vi "UI_uncorrupted.vi"() -> ()   [LabVIEW 2012]
doc: "Host interface for communication with CRD and PAS. This application currently must be running before the servers (PAS and CRD chassis) are running). At startup, the host will poll the LAN for a UDP connection to each instrument, pinging on port 5555. The acquisition loop will configure the FP and then move into a waiting state where it is polling for a connection on TCP/IP using the STM Connection Manager. When one of the instruments responds to the host, a new TCP connection will be opened on port 5556 and added to the connection manager. Seeing the connection, this VI will move from a wait state to the acquisition state where connections will be monitored. \n\nDuring the acquisition state, the host will handle messages sent via TCP/IP from the instruments. A queued state machine will determine how the data packets sent from the different instruments is handled."
uses:
  Interface/Controls/Host_State.ctl
  <vilib>/real-time/NI_Real-Time Libraries.lvlib
  Reusable/Xctls/Buffer/2D Control/2D Buffer Display.xctl
  Interface/CRDS/tau_state.ctl
  <vilib>/real-time/rtutility.llb/RT Restart Target (IP).vi
  Interface/Controls/PAS_MFC_SP.ctl
  Reusable/File IO/File Utilities.lvlib
  <userlib>/_JGCODE/error_logger/_error_logger.llb/ErrorLogger.lvclass
  Interface/CRDS/Controls/Ringdown Xctl/Ringdown.xctl
  Data/cPAS Cell Data/cPAS Cell Data.lvclass
  Data/cPAS Data.lvclass
  CRDS/Data/cCRDS Data.lvclass
  Reusable/PAS/Data/Cell/PAS Cell Data.lvclass
  Reusable/CRDS/Data/Cell/CRDS Cell Data.lvclass
  Interface/Controls/pasCellTEC.ctl
  Interface/Controls/pasTECen.ctl
  Interface/Controls/pasLasCtl.ctl
  Reusable/PAS/Main/Controls/Laser Modulation.ctl
  Utilities/FPGA/Controls/FPGAConfig.ctl
panel:
  in  "swDispl":T1
  in  "tabCtl":T2(tab)=enum."PAS Ctl"
  out "pasDerData":cluster{"data_out":sgl[][], "time":timestamp}(xcontrol)
  out "extWvfm":cluster{"data_out":sgl[][], "time":timestamp}(xcontrol)
  in  "crd::tec::en":cluster{"med":bool, "high":bool} caption="TEC Enable"
  in  "lasEn":T3
  out "TRHin":cluster{"hum":sgl, "dry":sgl} caption="Humidifier \nTemperatures (degC)" {"dry" format="%#.2f"; "hum" format="%#.2f"}
  in  "crd::rh":cluster{"hum":sgl, "dry":sgl} caption="Humidifier RH (%)" {"dry" format="%#.2f"; "hum" format="%#.2f"}
  in  "crd::rhctl":bool
  in  "crd::tec::T":cluster{"hum":sgl, "dry":sgl} caption="Humidifier \nTemperatures (degC)" {"dry" format="%#.2f"; "hum" format="%#.2f"}
  out "vaisalaData":T4 caption="Vaisala Data" {"ref 2"."TRH" format="%.2f"; "ref 2"."RH" format="%.2f"; "ref"."TRH" format="%.2f"; "ref"."RH" format="%.2f"; "dry"."TRH" format="%.2f"; "dry"."RH" format="%.2f"; "hum"."TRH" format="%.2g"; "hum"."RH" format="%.2g"}
  out "alctData":T5 caption="Alicat Data" {"purge"."P" format="%.2f"; "purge"."T" format="%.2f"; "purge"."Q" format="%.2f"; "hRH"."P" format="%.2f"; "hRH"."T" format="%.2f"; "hRH"."Q" format="%.2f"; "mRH"."P" format="%.2f"; "mRH"."T" format="%.2f"; "mRH"."Q" format="%.2f"; "dry"."P" format="%.2f"; "dry"."T" format="%.2f"; "dry"."Q" format="%.2f"; "denude"."P" format="%.2f"; "denude"."T" format="%.2f"; "denude"."Q" format="%.2f"}
  out "P":T6 caption="Pressure (mb)" {"ref 2" format="%#.2f"; "ref" format="%#.2f"; "dry" format="%#.2f"; "hum" format="%#.2f"}
  in  "Laser Controls":cluster{"f (Hz)":dbl, "Duty Cycle (%)":dbl}
  in  "crdFlows":T7 caption="Flow Rate Setpoints (LPM)" {"purge" max=5 format="%.2f"; "hRH" max=5 format="%.2f"; "mRH" max=5 format="%.2f"; "dry" max=5 format="%.2f"; "denude" max=5 format="%.2f"}
  in  "pasLasCtl":T8 caption="Laser Control" {"Laser Output"."Span"."ch 5" min=0 max=20; "Laser Output"."Span"."ch 4" min=0 max=20; "Laser Output"."Span"."ch 3" min=0 max=20; "Laser Output"."Span"."ch 2" min=0 max=20; "Laser Output"."Span"."ch 1" min=0 max=20; "f0"."Cell 1" max=2000 step=1; "f0"."Cell 2" max=2000 step=1; "f0"."Cell 3" max=2000 step=1; "f0"."Cell 4" max=2000 step=1; "f0"."Cell 5" max=2000 step=1}
  out "PASCellT2":T11 caption="Thermistor Cell Temperature (degC)" {"Cell 5" format="%.2f"; "Cell 4" format="%.2f"; "Cell 3" format="%.2f"; "Cell 2" format="%.2f"; "Cell 1" format="%.2f"}
  out "tecP":sgl caption="TEC Power (%)" format="%#.2f"
  in  "pas::rhctl":bool caption="RH Control"
  in  "pas::rh":dbl caption="RH (%)"
  in  "ptecHumEn":bool caption="Enable"
  in  "pas::satT":sgl caption="T(degC)"
  out "PASCellT":T12 caption="TEC Thermistor Cell Temperature (degC)" {"Cell 5" format="%.2f"; "Cell 4" format="%.2f"; "Cell 3" format="%.2f"; "Cell 2" format="%.2f"; "Cell 1" format="%.2f"}
  out "pasRH":T13 caption="Vaisala Data" {"c 5"."TRH" format="%#.2f"; "c 5"."RH" format="%#.2f"; "c 4"."TRH" format="%#.2f"; "c 4"."RH" format="%#.2f"; "c 3"."TRH" format="%#.2f"; "c 3"."RH" format="%#.2f"; "c 2"."TRH" format="%#.2f"; "c 2"."RH" format="%#.2f"; "c 1"."TRH" format="%#.2f"; "c 1"."RH" format="%#.2f"}
  out "pasACat":T14 caption="Alicat Data" {"c 5 2"."P" format="%.2f"; "c 5 2"."T" format="%.2f"; "c 5 2"."Q" format="%.2f"; "c 4"."P" format="%.2f"; "c 4"."T" format="%.2f"; "c 4"."Q" format="%.2f"; "c 3"."P" format="%.2f"; "c 3"."T" format="%.2f"; "c 3"."Q" format="%.2f"; "c 2"."P" format="%.2f"; "c 2"."T" format="%.2f"; "c 2"."Q" format="%.2f"; "c 1"."P" format="%.2f"; "c 1"."T" format="%.2f"; "c 1"."Q" format="%.2f"}
  out "pasTte":sgl caption="TEC Temperature\n(degC)" format="%#.2f"
  in  "pasTECEn":T15 caption="Enable TECs"
  in  "pasTcell":T16 caption="Temperature \n (degC)"
  in  "pasFlows":T17 caption="Flow Rate Setpoint (LPM)" {"Cell 5" min=0 max=5; "Cell 4" min=0 max=5; "Cell 3" min=0 max=5; "Cell 2" min=0 max=5; "Cell 1" min=0 max=5}
  in  "pasTteSP":sgl caption="TEC Temperature \nSetpoint (degC)" format="%#.2f"
  out "Thum":sgl caption="Tsat\n(degC)" format="%#.2g"
  out "pasHK":cluster{"data_out":sgl[][], "time":timestamp}(xcontrol)
  out "crdHK":cluster{"data_out":sgl[][], "time":timestamp}(xcontrol)
  out "Ringdown":i16[][][](xcontrol)
  in  "log_lin":bool
  out "Q":sgl format="%.2f"
  out "f0":sgl
  in  "cell":T18(ring)
  out "micTime":waveform(i16)(graph) caption="Time Domain"
  out "micFreq":cluster{i32, dbl, "Y":sgl[]}[](graph) caption="Frequency Domain"
  out "diodeTime":waveform(i16)(graph) caption="Photodiode Time Domain"
  out "lastCal":timestamp caption="Last Speaker Calibration" format="%<%H:%M:%S>T"
  in  "filtSpot":u8 caption="Filter Spot" max=8 step=1
  out "O3Q":cluster{"Q":sgl, "T":sgl, "P":sgl} caption="Alicat Data" {"P" format="%.2f"; "T" format="%.2f"; "Q" format="%.2f"}
  in  "QO3":sgl caption="Flow Rate \n(sccm)"
  in  "O3 level":u8(slide) max=10 step=1 scale=0.0..5.0
  out "clapQ":cluster{"Q":sgl, "T":sgl, "P":sgl} caption="Alicat Data" {"P" format="%.2f"; "T" format="%.2f"; "Q" format="%.2f"}
  in  "Qclap":sgl caption="Flow Rate \n(lpm)"
  out "clapData":string caption="Data Stream"
  in  "ACpow":T19
  out "dcVolts":T20 caption="DC Power Supply" {"Aux" format="%#.2g"; "12 V" format="%#.2g"; "-15 V" format="%#.2g"; "+15 V" format="%#.2g"; "24 V" format="%#.2g"}
  in  "spk_en":bool
  out "rdError":bool caption="RD Error"
  out "pasComm":bool
  out "crdComm":bool
  out "genError":bool caption="General Error"
  out "filtTime":timestamp caption="Last Filter Switch" format="%<%H:%M:%S>T"
  out "pasTime":timestamp caption="PAS Time" format="%<%H:%M:%S>T"
  out "uDrive":bool caption="U drive?"
  out "bypass?":bool caption="Bypass?"
  in  "bypass":bool
  out "filter?":bool caption="Filter?"
  out "crdTime":timestamp caption="CRD Time" format="%<%H:%M:%S>T"
  in  "filter":bool
  out "svRDs":bool caption="Saving Ringdowns"
  out "write":bool caption="Writing Data"
  out "crdError":bool caption="CRDS Error"
  out "pasErr":bool caption="PAS Error"
  out "pasSpk":bool caption="PAS Speaker On?"
  # "CRD Controls"
  # "CRD Controller Data"
  # "Laser Enable"
  # "PAS Controls"
  # "PAS Housekeeping Data"
  # "TEC Temperature Control"
  # "RH Control"
  # "Power"
  # "CLAP"
  # "To turn on the CLAP, use AC 2 above."
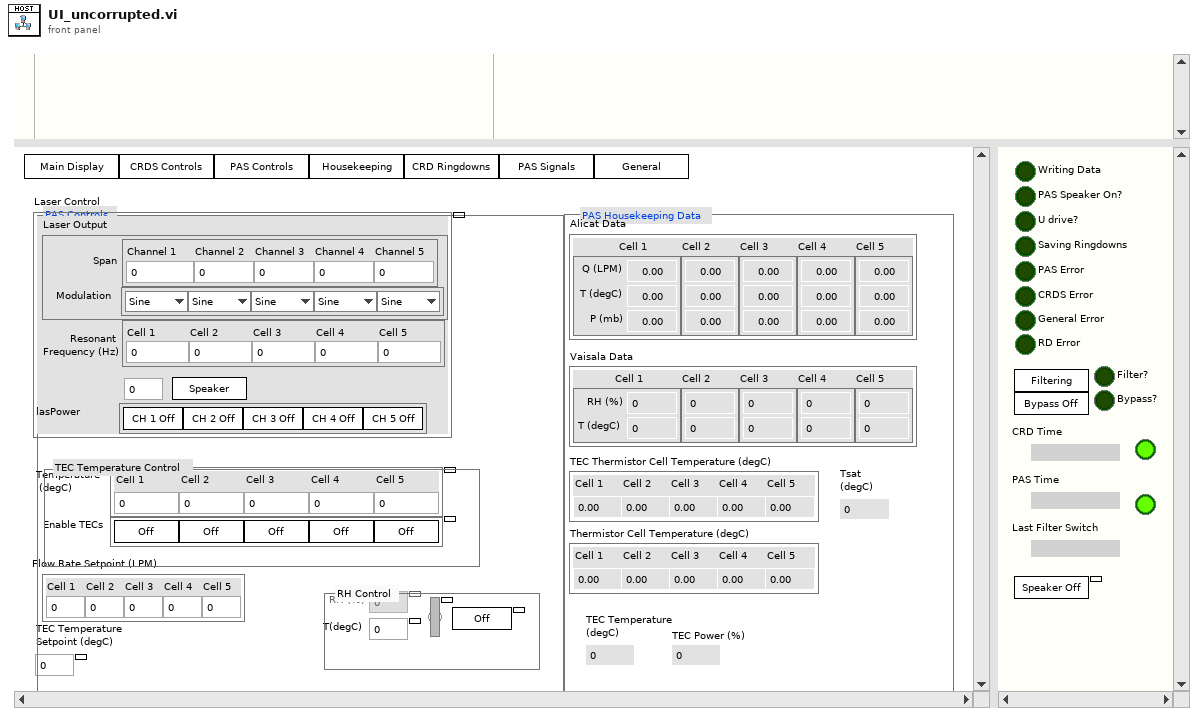
[diagram p1: front panel]
types:
  T1 = cluster{"mDispl":bool, "crdCtl":bool, "pasCtl":bool, "housekeeping":bool, "crdRD":bool, "pasSig":bool, "power":bool}
  T2 = enum32{"main", "CRDCtl", "PAS Ctl", "housekeeping", "crdRD", "pasSig", "power"}
  T3 = cluster{"red":bool, "Blue":bool, "Aux":bool, "Green":bool}
  T4 = cluster{"hum":cluster{"RH":sgl, "TRH":sgl}, "dry":cluster{"RH":sgl, "TRH":sgl}, "ref":cluster{"RH":sgl, "TRH":sgl}, "ref 2":cluster{"RH":sgl, "TRH":sgl}}
  T5 = cluster{"denude":cluster{"Q":sgl, "T":sgl, "P":sgl}, "dry":cluster{"Q":sgl, "T":sgl, "P":sgl}, "mRH":cluster{"Q":sgl, "T":sgl, "P":sgl}, "hRH":cluster{"Q":sgl, "T":sgl, "P":sgl}, "purge":cluster{"Q":sgl, "T":sgl, "P":sgl}}
  T6 = cluster{"hum":sgl, "dry":sgl, "ref":sgl, "ref 2":sgl}
  T7 = cluster{"denude":sgl, "dry":sgl, "mRH":sgl, "hRH":sgl, "purge":sgl}
  T8 = typedef "pasLasCtl.ctl" = cluster{"Laser Output":T9, "f0":cluster{"Cell 1":u16, "Cell 2":u16, "Cell 3":u16, "Cell 4":u16, "Cell 5":u16}, "drive":bool, "Speake Voltage":sgl, "lasPower":cluster{"ch 1":bool, "ch 2":bool, "ch 3":bool, "ch 4":bool, "ch 5":bool}}
  T9 = typedef "FPGAConfig.ctl" = cluster{"Span":cluster{"ch 1":sgl, "ch 2":sgl, "ch 3":sgl, "ch 4":sgl, "ch 5":sgl}, "mod":cluster{"ch 1":T10, "ch 2":T10, "ch 3":T10, "ch 4":T10, "ch 5":T10}}
  T10 = typedef "Laser Modulation.ctl" = enum8{"Sine", "Square"}
  T11 = cluster{"[0]":sgl, "[1]":sgl, "[2]":sgl, "[3]":sgl, "[4]":sgl}
  T12 = cluster{"ScaledData[0]":sgl, "ScaledData[1]":sgl, "ScaledData[2]":sgl, "ScaledData[3]":sgl, "ScaledData[4]":sgl}
  T13 = cluster{"c 1":cluster{"RH":sgl, "TRH":sgl}, "c 2":cluster{"RH":sgl, "TRH":sgl}, "c 3":cluster{"RH":sgl, "TRH":sgl}, "c 4":cluster{"RH":sgl, "TRH":sgl}, "c 5":cluster{"RH":sgl, "TRH":sgl}}
  T14 = cluster{"c 1":cluster{"Q":sgl, "T":sgl, "P":sgl}, "c 2":cluster{"Q":sgl, "T":sgl, "P":sgl}, "c 3":cluster{"Q":sgl, "T":sgl, "P":sgl}, "c 4":cluster{"Q":sgl, "T":sgl, "P":sgl}, "c 5 2":cluster{"Q":sgl, "T":sgl, "P":sgl}}
  T15 = typedef "pasTECen.ctl" = cluster{"Cell 1":bool, "Cell 2":bool, "Cell 3":bool, "Cell 4":bool, "Cell 5":bool}
  T16 = typedef "pasCellTEC.ctl" = cluster{"Cell 1":sgl, "Cell 2":sgl, "Cell 3":sgl, "Cell 4":sgl, "Cell 5":sgl}
  T17 = typedef "PAS_MFC_SP.ctl" = cluster{"Cell 1":sgl, "Cell 2":sgl, "Cell 3":sgl, "Cell 4":sgl, "Cell 5":sgl}
  T18 = enum16{"Cell 1", "Cell 2", "Cell 3", "Cell 4", "Cell 5"}
  T19 = cluster{"ac1 2":bool, "ac1 3":bool, "ac1":bool, "ac2":bool, "ac3":bool, "O3":bool, "wp1":bool, "wp2":bool}
  T20 = cluster{"24 V":dbl, "+15 V":dbl, "-15 V":dbl, "12 V":dbl, "Aux":dbl}
  T21 = typedef "Host_State.ctl" = enum16{"Config", "Acquire", "Write CRD Data", "Write PAS Data", "Chk PAS Flt", "Chk CRD Flt", "O3 Calibration", "Check AO Queue", "Error", "Wait", "Quit", "Disconnect"}
  T22 = enum32{"invalid app kind", "Development System", "Run Time System", "Student Edition", "Embedded LabVIEW", "Evaluation", "Custom"}
  T23 = enum8{"Enabled", "Disabled", "Disabled and Grayed Out"}
  T24 = typedef "tau_state.ctl" = enum16{"Config", "Write", "Close"}
  T25 = cluster{"ACPow[0]":bool, "ACPow[1]":bool, "ACPow[2]":bool, "ACPow[3]":bool, "ACPow[4]":bool, "ACPow[5]":bool, "ACPow[6]":bool, "ACPow[7]":bool}
  T26 = cluster{"Numeric":sgl, "Numeric":sgl, "Numeric":sgl}
  T27 = cluster{"24V":sgl, "+15V":sgl, "- 15V":sgl, "12V":sgl, "Aux Volt":sgl}
  T28 = cluster{"[0]":cluster{"Q":sgl, "T":sgl, "P":sgl}, "[1]":cluster{"Q":sgl, "T":sgl, "P":sgl}, "[2]":cluster{"Q":sgl, "T":sgl, "P":sgl}, "[3]":cluster{"Q":sgl, "T":sgl, "P":sgl}, "[4]":cluster{"Q":sgl, "T":sgl, "P":sgl}}
  T29 = cluster{"Input 1":sgl, "Input 2":sgl, "Power":sgl}
  T30 = cluster{"f0":sgl, "IA":sgl, "Q":sgl, "max":dbl[], "deltaPhi":dbl, "tau":dbl, "noiseLim":dbl, "ext":dbl}
  T31 = cluster{"f0":sgl, "IA":sgl, "Q":sgl, "max":sgl[], "deltaPhi":sgl, "tau":sgl, "noiseLim":sgl, "ext":sgl}
  T32 = cluster{"T":sgl, "TRH":sgl, "RH":sgl, "laserRMS":sgl}
  T33 = cluster{"[0]":cluster{"RH":sgl, "TRH":sgl}, "[1]":cluster{"RH":sgl, "TRH":sgl}, "[2]":cluster{"RH":sgl, "TRH":sgl}, "[3]":cluster{"RH":sgl, "TRH":sgl}, "[4]":cluster{"RH":sgl, "TRH":sgl}}
  T34 = cluster{"P":sgl, "T":sgl, "Q":sgl, "Q0":sgl, "Qsp":sgl}[]
  T35 = cluster{"Array of Single[0]":sgl, "Array of Single[1]":sgl}
  T36 = cluster{"Pressure[0]":sgl, "Pressure[1]":sgl, "Pressure[2]":sgl, "Pressure[3]":sgl}
  T37 = cluster{"vData[0]":cluster{"TRH":dbl, "RH":dbl}, "vData[1]":cluster{"TRH":dbl, "RH":dbl}, "vData[2]":cluster{"TRH":dbl, "RH":dbl}, "vData[3]":cluster{"TRH":dbl, "RH":dbl}}
  T38 = typedef "extparam.ctl" = cluster{"Tau":sgl, "Tau0cor":sgl, "ext":sgl, "extCorr":sgl, "stdevTau":sgl, "eTau":sgl, "taucorr":sgl, "Tau0":sgl, "max":sgl}
  T39 = typedef "calData.ctl" = cluster{"rhDilFac":sgl, "Q":sgl, "Tmean":sgl, "extDilFac":sgl, "rhCell":sgl, "P":sgl, "T":sgl}
  T40 = cluster{"Data Access:extParam":sgl[][], "Time":timestamp}
  T41 = cluster{"P":sgl, "T":sgl, "Q":sgl, "Q0":sgl, "Qsp":sgl}
  T42 = cluster{"c 1":bool, "c 2":bool, "c 3":bool, "c 4":bool, "c 5":bool}
  T43 = cluster{"Name":string, "Line Width":u8, "Line Style":u8, "Color":u32}[]
  T44 = cluster{"[0]":bool, "[1]":bool, "[2]":bool, "[3]":bool, "[4]":bool, "[5]":bool, "[6]":bool}
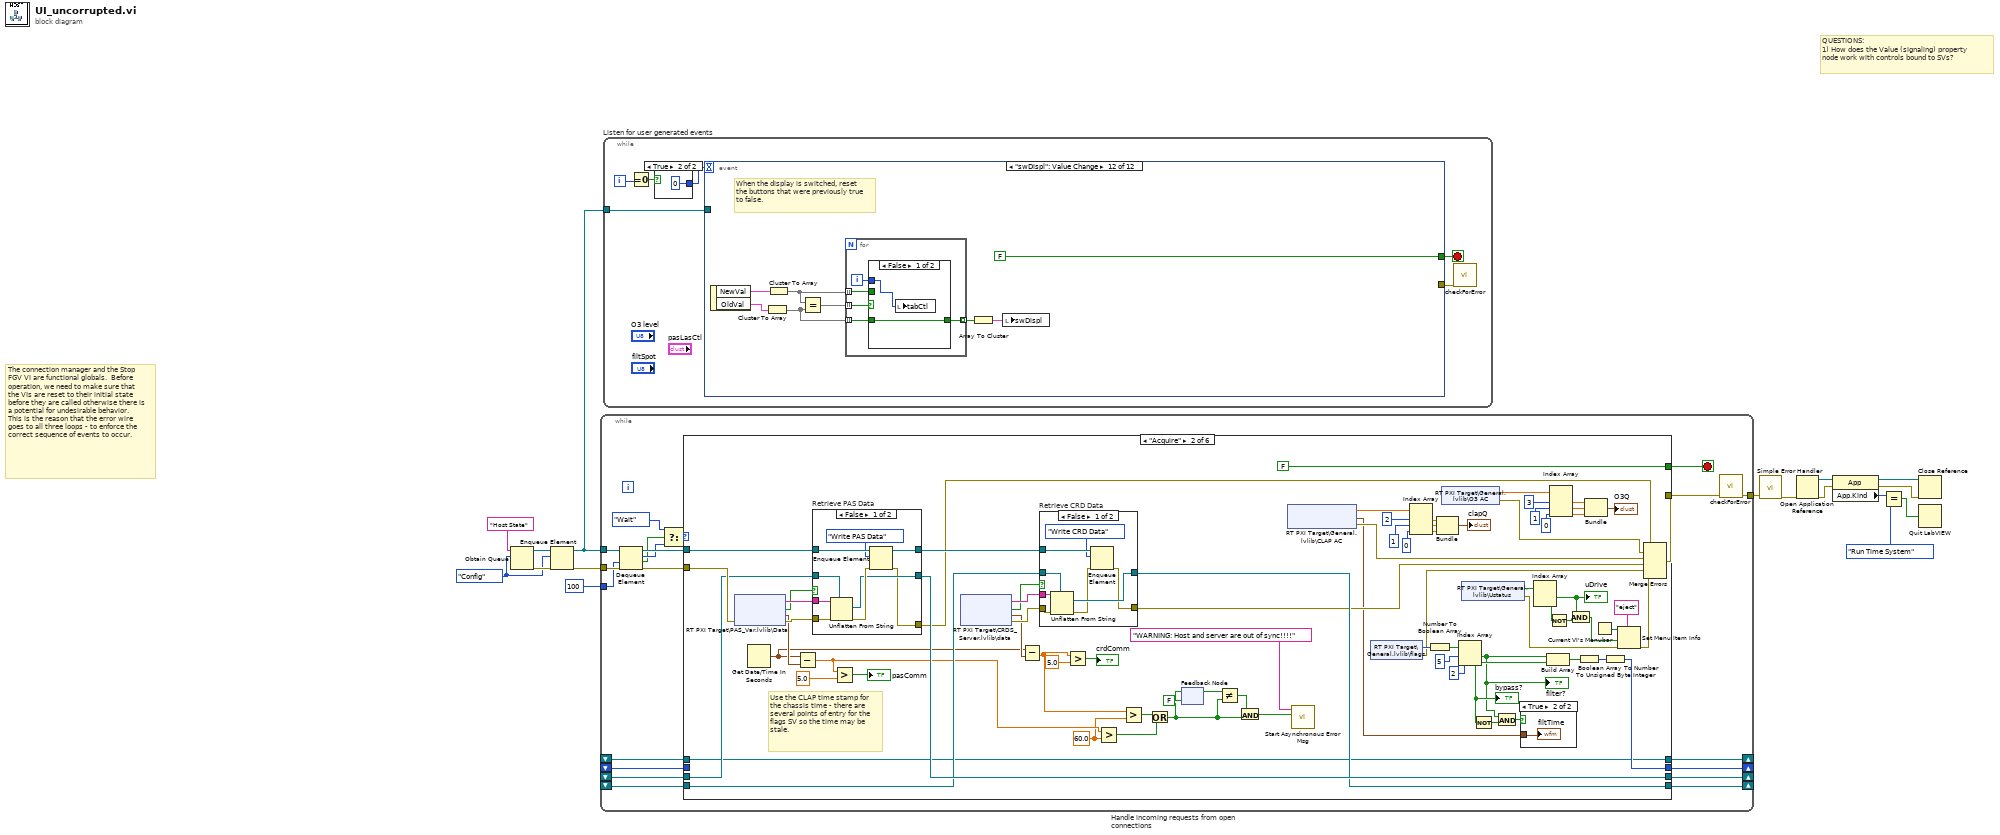
[diagram p0: block diagram]
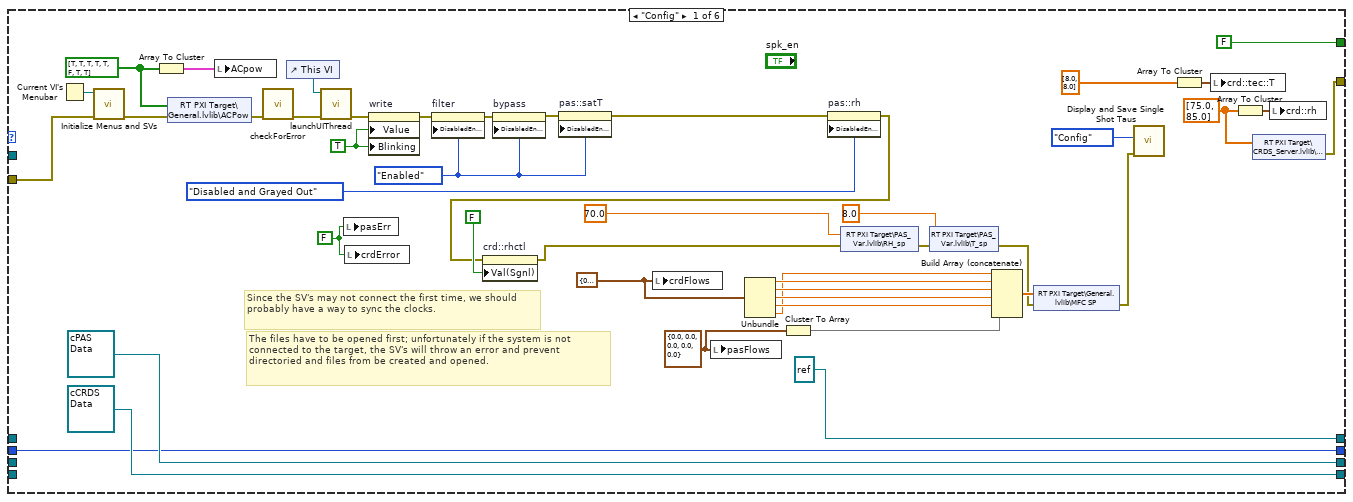
[diagram p2: hidden frame]
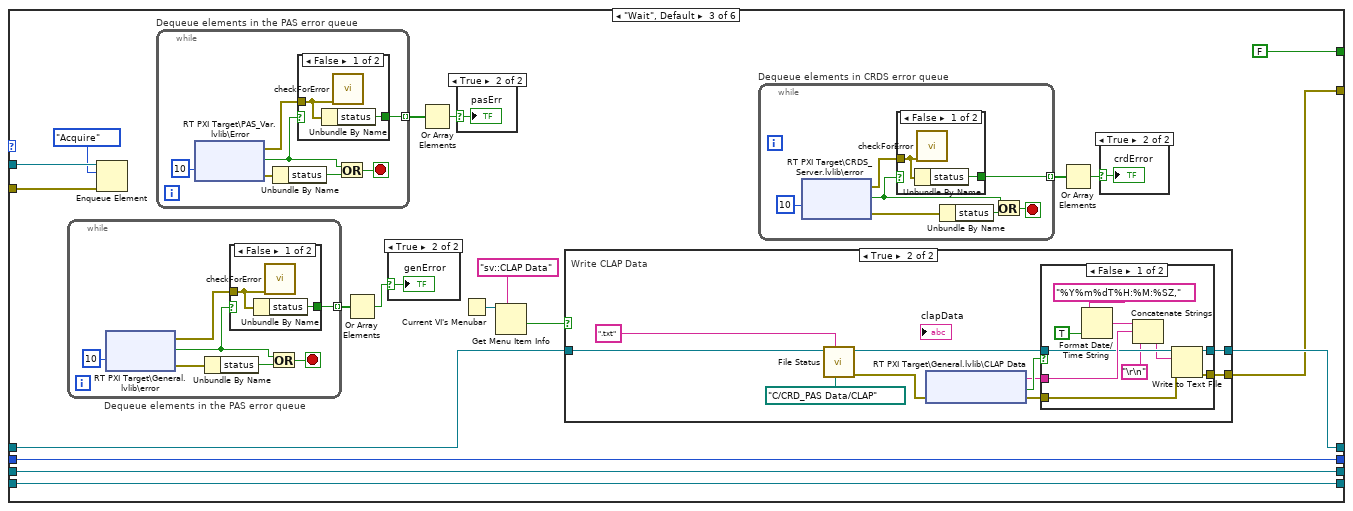
[diagram p6: hidden frame]
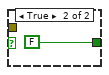
[diagram p8: hidden frame]
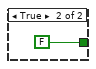
[diagram p13: hidden frame]
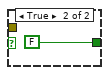
[diagram p14: hidden frame]
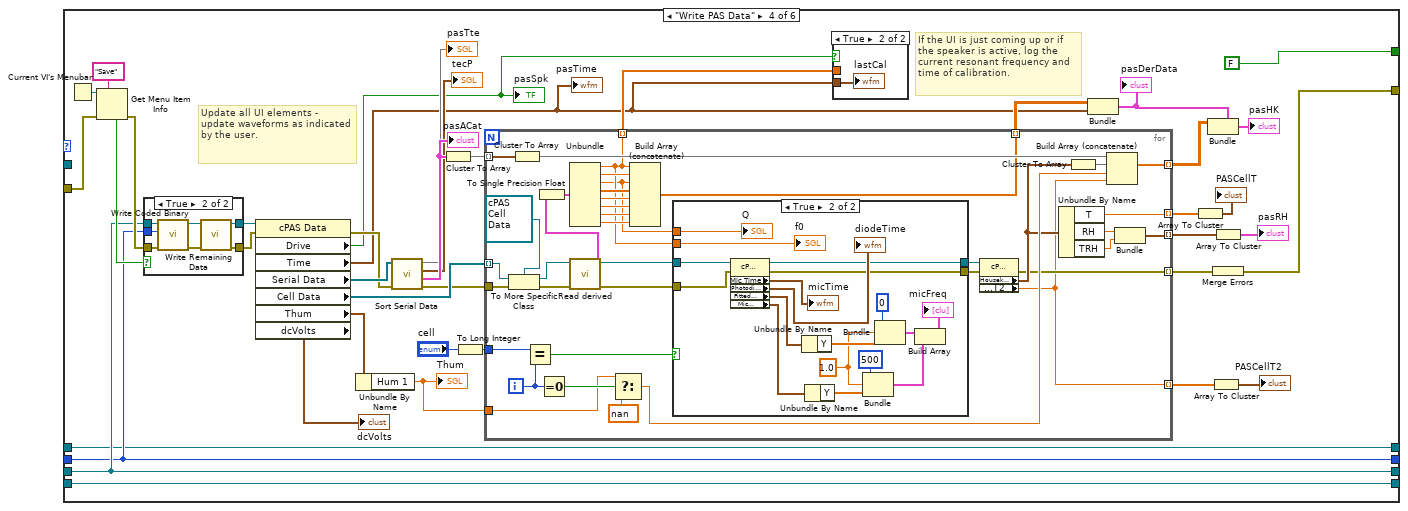
[diagram p15: hidden frame]
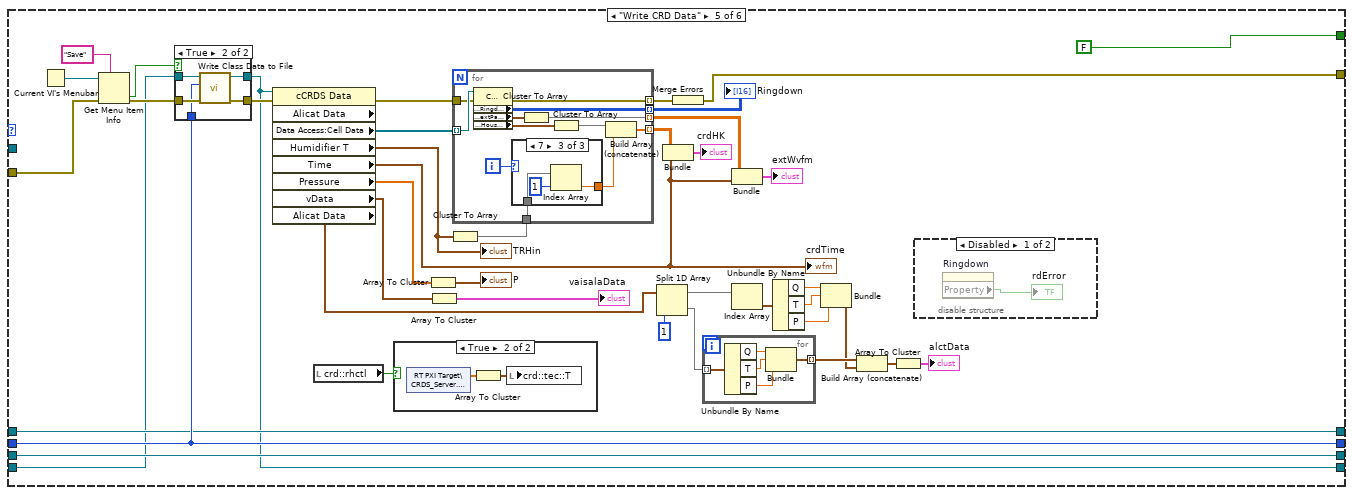
[diagram p19: hidden frame]
diagram:
  w5 = Host_State."Config" ("Host_State")
  # "QUESTIONS:\n1) How does the Value (signaling) property node work with controls bound to SVs?"
  # "The connection manager and the Stop FGV VI are functional globals.  Before operation, we need to make sure that the VIs are reset to their initial state before they are called otherwise there is a potential for undesirable behavior.  This is the reason that the error wire goes to all three loops - to enforce the correct sequence of events to occur."
  n1 = Obtain Queue(name (unnamed)="Host State", element data type=w5) -> (queue out=w7:refnum<queue>, error out=w6:errorcluster)  [unwired: 3 in, 1 out]
  n2 = Enqueue Element(queue=w7, element=w5, error in (no error)=w6) -> (queue out=w2:refnum<queue>, error out=w1:errorcluster)  [unwired: 1 in, 1 out]
  n3 = while "Handle incoming requests from open connections" {
    tunnel: w2 -> [w36]
    tunnel: w1 -> [w34]
    tunnel: [w17] -> w3
    tunnel: 100 ("timeout in ms (-1)") -> [w27]
    shift-right: [w26] -> _
    shift-left: _ -> [w25]
    shift-right: [w24] -> _
    shift-left: _ -> [w23]
    shift-right: [w22] -> _
    shift-left: _ -> [w21]
    shift-right: [w20] -> _
    shift-left: _ -> [w19]
    stop <- w32 stop-if-true
    n4 = Dequeue Element(queue=w36, timeout in ms (-1)=w27, error in (no error)=w34) -> (queue out=w35:refnum<queue>, element=w31:T21, timed out?=w29:bool, error out=w33:errorcluster)
    n5 = Select(t=Host_State."Wait", s=w29, f=w31) -> (s? t:f=w28:T21)
    n6 = case shown="\"Acquire\"" w28 {
      tunnel: w33 -> [w78 w155 w194 w278 w382 w469]
      tunnel: w35 -> [_ w153 w198 _ _ w470]
      tunnel: [FALSE FALSE FALSE FALSE FALSE TRUE] -> w32
      tunnel: [refnum<class "cPAS Data.lvclass"> refnum ("PAS Data.lvclass") w154 w199 w269 w404 refnum<class "cPAS Data.lvclass"> refnum ("cPAS Data")] -> w26
      tunnel: w25 -> [_ w151 w199 w269 w404 _]
      tunnel: [w49 w134 w183 w279 w373 w453] -> w18
      tunnel: [refnum<class "cCRDS Data.lvclass"> refnum ("cPAS Library.lvlib:cCRDS Data") w147 w192 w276 w364 refnum<class "cCRDS Data.lvclass"> refnum ("cPAS Library.lvlib:cCRDS Data")] -> w24
      tunnel: w23 -> [_ w149 w192 w276 w365 _]
      tunnel: [w72 w132 w191 w266 w372 w447] -> w22
      tunnel: w21 -> [w72 _ w191 w266 w372 w447]
      tunnel: [refnum<file> refnum ("fileRefOut") w121 w190 w265 w369 refnum<file> refnum ("fileRefOut")] -> w20
      tunnel: w19 -> [_ w121 w189 w265 w369 w443]
      frame "Config" {
        w48 = FALSE
        w51 = sgl[] [75.0, 85.0] ("RHsp")
        w58 = T17 {"Cell 1"=0.0, "Cell 2"=0.0, "Cell 3"=0.0, "Cell 4"=0.0, "Cell 5"=0.0} ("pasFlows")
        w59 = T7 {"denude"=0.0, "dry"=0.0, "mRH"=0.0, "hRH"=0.0, "purge"=0.16} ("crdFlows")
        w41 = T23."Enabled" ("Disabled")
        w76 = TRUE
        w77 = bool[] [TRUE, TRUE, TRUE, TRUE, TRUE, FALSE, TRUE, TRUE] ("ACPow")
        # "Since the SV's may not connect the first time, we should probably have a way to sync the clocks."
        # "The files have to be opened first; unfortunately if the system is not connected to the target, the SV's will throw an error and prevent directoried and files from be created and opened."
        n7 = Current VI's Menubar() -> (w79:refnum<k9>)
        n8 = call "Initialize Menus and SVs.vi"("error in"=w78, "Menu in"=w79) -> ("error out"=w68:errorcluster)  [unwired: 9 in]
        n9 = Array To Cluster(array=w77) -> (cluster=w73:T25)
        n10 = shared-variable "RT PXI Target\\General.lvlib\\ACPow"(w77, error in=w68) -> (error out=w46:errorcluster)
        n11 = local write "ACpow"(w73) -> ()
        n12 = call <userlib>:"checkForError.vi"("Error In"=w46) -> ("error out"=w45:errorcluster)  [unwired: 9 in, 1 out]
        n13 = control-ref of="This VI"() -> (w44:refnum<vi>)
        n14 = call <userlib>:"launchUIThread.vi"("error in (no error)"=w45, "UI VI Refnum"=w44) -> ("error out"=w47:errorcluster)  [unwired: 9 in]
        n15 = local write "pasErr"(w48) -> ()
        n16 = local write "crdError"(w48) -> ()
        n17 = property on="write" class="Bool (strict)"(error in=w47, "Value"=w76, "Blinking"=w76) -> (error out=w67:errorcluster)  [unwired: 1 in, 1 out]
        n18 = property on="filter" class="Bool (strict)"(error in=w67, "DisabledEnum"=w41) -> (error out=w69:errorcluster)  [unwired: 1 in, 1 out]
        n19 = property on="bypass" class="Bool (strict)"(error in=w69, "DisabledEnum"=w41) -> (error out=w42:errorcluster)  [unwired: 1 in, 1 out]
        n20 = property on="pas::satT" class="DigNum (strict)"(error in=w42, "DisabledEnum"=w41) -> (error out=w40:errorcluster)  [unwired: 1 in, 1 out]
        n21 = local write "crdFlows"(w59) -> ()
        n22 = local write "pasFlows"(w58) -> ()
        n23 = Unbundle(w59) -> ("denude"=w61:sgl, "dry"=w62:sgl, "mRH"=w63:sgl, "hRH"=w64:sgl, "purge"=w60:sgl)
        n24 = Cluster To Array(cluster=w58) -> (array=w65:sgl[])
        n25 = property on="pas::rh" class="DigNum (strict)"(error in=w40, "DisabledEnum"=T23."Disabled and Grayed Out" ("Disabled")) -> (error out=w39:errorcluster)  [unwired: 1 in, 1 out]
        n26 = property on="crd::rhctl" class="Bool (strict)"(error in=w39, "Val(Sgnl)"=FALSE ("RHctl?")) -> (error out=w37:errorcluster)  [unwired: 1 in, 1 out]
        n27 = shared-variable "RT PXI Target\\PAS_Var.lvlib\\RH_sp"(sgl 70.0 ("RH_sp"), error in=w37) -> (error out=w55:errorcluster)
        n28 = shared-variable "RT PXI Target\\PAS_Var.lvlib\\T_sp"(sgl 8.0 ("T_sp"), error in=w55) -> (error out=w38:errorcluster)
        n29 = Build Array (concatenate)(w60, w61, w62, w63, w64, w65) -> (w66:sgl[])
        n30 = shared-variable "RT PXI Target\\General.lvlib\\MFC SP"(w66, error in=w38) -> (error out=w53:errorcluster)
        n31 = call "Display and Save Single Shot Taus.vi"("error in"=w53, "state"=tau_state."Config") -> ()  [unwired: 9 in, 1 out]
        n32 = Array To Cluster(array=sgl[] [8.0, 8.0] ("ThumSP")) -> (cluster=w70:cluster{"ThumSP[0]":sgl, "ThumSP[1]":sgl})
        n33 = local write "crd::tec::T"(w70) -> ()
        n34 = Array To Cluster(array=w51) -> (cluster=w50:cluster{"RHsp[0]":sgl, "RHsp[1]":sgl})
        n35 = shared-variable "RT PXI Target\\CRDS_Server.lvlib\\RHsp"(w51) -> (error out=w49:errorcluster)  [unwired: 1 in]
        n36 = local write "crd::rh"(w50) -> ()
      }
      frame "Acquire" {
        w90 = 60.0 ("y")
        # "Use the CLAP time stamp for the chassis time - there are several points of entry for the flags SV so the time may be stale."
        n37 = shared-variable "RT PXI Target\\PAS_Var.lvlib\\Data"(error in=w155) -> (w156:string, error out=w157:errorcluster, w144:bool, w99:timestamp)  [unwired: 1 in]
        n38 = Get Date/Time In Seconds() -> (seconds since 1Jan1904=w94:timestamp)
        n39 = Subtract(x=w94, y=w99) -> (x-y=w91:dbl)
        n40 = case "Retrieve PAS Data" shown="False" w144 {
          tunnel: w157 -> [w177 w178]
          tunnel: w156 -> [w176 _]
          tunnel: [w170 w179] -> w154
          tunnel: w153 -> [w175 w180]
          tunnel: w151 -> [w171 w179]
          tunnel: [w174 w180] -> w150
          tunnel: [w169 w178] -> w131
          frame False {
            n41 = Unflatten From String(type=w171, binary string=w176, error in (no error)=w177) -> (value=w170:refnum<class "cPAS Data.lvclass">, error out=w172:errorcluster)  [unwired: 2 in, 1 out]
            n42 = Enqueue Element(queue=w175, element=Host_State."Write PAS Data", error in (no error)=w172) -> (queue out=w174:refnum<queue>, error out=w169:errorcluster)  [unwired: 1 in, 1 out]
          }
          frame True {
          }
        }
        n43 = Greater?(x=w91, y=5.0) -> (0:→"pasComm":bool)
        n44 = shared-variable "RT PXI Target\\CRDS_Server.lvlib\\data"() -> (w146:string, error out=w148:errorcluster, w143:bool, w95:timestamp)  [unwired: 2 in]
        n45 = Subtract(x=w94, y=w95) -> (x-y=w92:dbl)
        n46 = case "Retrieve CRD Data" shown="False" w143 {
          tunnel: w150 -> [w166 _]
          tunnel: w149 -> [w165 w168]
          tunnel: w148 -> [w164 w167]
          tunnel: [w163 w168] -> w147
          tunnel: [w162 w167] -> w135
          tunnel: w146 -> [w161 _]
          frame False {
            n47 = Unflatten From String(type=w165, binary string=w161, error in (no error)=w164) -> (value=w163:refnum<class "cCRDS Data.lvclass">, error out=w159:errorcluster)  [unwired: 2 in, 1 out]
            n48 = Enqueue Element(queue=w166, element=Host_State."Write CRD Data", error in (no error)=w159) -> (error out=w162:errorcluster)  [unwired: 1 in, 2 out]
          }
          frame True {
          }
        }
        n49 = Greater?(x=w92, y=5.0) -> (0:→"crdComm":bool)
        n50 = Greater?(x=w91, y=w90) -> (0:w88:bool)
        n51 = Greater?(x=w92, y=w90) -> (0:w89:bool)
        n52 = Or(x=w89, y=w88) -> (x .or. y?=w82:bool)
        n53 = feedback-in #1(w82) -> ()
        n54 = feedback #1(FALSE) -> (w83:bool)
        n55 = Not Equal?(x=w83, y=w82) -> (x != y?=w87:bool)
        n56 = And(x=w87, y=w82) -> (x .and. y?=w86:bool)
        n57 = shared-variable "RT PXI Target\\General.lvlib\\CLAP AC"() -> (w129:sgl[], error out=w130:errorcluster, w104:timestamp)  [unwired: 1 in]
        n58 = call "Start Asynchronous Error Msg.vi"("throw msg?"=w86, "eMsg"="WARNING: Host and server are out of sync!!!!") -> ()  [unwired: 9 in, 1 out]
        n59 = shared-variable "RT PXI Target\\General.lvlib\\flags"() -> (w120:u8, error out=w107:errorcluster)  [unwired: 1 in]
        n60 = Index Array(array=w129, index #1=2 ("index"), index #2=1 ("index"), index #3=0 ("index")) -> (element #1=w125:sgl, element #2=w124:sgl, element #3=w123:sgl)
        n61 = Number To Boolean Array(number=w120) -> (Boolean array=w119:bool[])
        n62 = Bundle("Numeric"=w125, "Numeric"=w124, "Numeric"=w123) -> (→"clapQ":T26)  [unwired: 1 in]
        n63 = shared-variable "RT PXI Target\\General.lvlib\\O3 AC"() -> (w110:sgl[], error out=w106:errorcluster)  [unwired: 1 in]
        n64 = Index Array(array=w119, index #1=5 ("index"), index #2=2 ("index")) -> (element #1=w100:bool, element #2=w102:bool)
        "filter?" <- w100
        "bypass?" <- w102
        n65 = shared-variable "RT PXI Target\\General.lvlib\\Ustatus"() -> (w142:bool[], error out=w105:errorcluster)  [unwired: 1 in]
        n66 = Not(x=w102) -> (.not. x?=w101:bool)
        n67 = And(x=w100, y=w101) -> (x .and. y?=w103:bool)
        n68 = case shown="True" w103 {
          tunnel: w104 -> [_ w158]
          frame False {
          }
          frame True {
            "filtTime" <- w158
          }
        }
        n69 = Index Array(array=w142) -> (element #1=w140:bool, element #2=w141:bool)  [unwired: 2 in]
        "uDrive" <- w140
        n70 = Build Array(w100, w102) -> (w145:bool[])
        n71 = Not(x=w141) -> (.not. x?=w139:bool)
        n72 = Index Array(array=w110, index #1=3 ("index"), index #2=1 ("index"), index #3=0 ("index")) -> (element #1=w114:sgl, element #2=w115:sgl, element #3=w116:sgl)
        n73 = And(x=w140, y=w139) -> (x .and. y?=w137:bool)
        n74 = Boolean Array To Number(Boolean array=w145) -> (number=w133:u32)
        n75 = Bundle("Numeric"=w114, "Numeric"=w115, "Numeric"=w116) -> (→"O3Q":T26)  [unwired: 1 in]
        n76 = Current VI's Menubar() -> (w138:refnum<k9>)
        n77 = To Unsigned Byte Integer(number=w133) -> (unsigned 8bit integer=w132:u8)
        n78 = Set Menu Item Info(7:"eject" ("item tag"), 8:w105, 9:w137, 11:w138) -> (0:w108:errorcluster)  [unwired: 3 in, 1 out]
        n79 = Merge Errors(w131, w106, w130, w135, w107, w108) -> (w134:errorcluster)
      }
      frame "Wait", Default {
        n80 = while "Dequeue elements in the PAS error queue" {
          tunnel: [w206] -> w182 mode=indexing
          stop <- w204 stop-if-true
          n81 = shared-variable "RT PXI Target\\General.lvlib\\error"(10 ("ms timeout (0)")) -> (w202:errorcluster, error out=w203:errorcluster, w201:bool)  [unwired: 1 in, 1 out]
          n82 = Unbundle By Name(w203) -> ("status"=w205:bool)
          n83 = case shown="False" w201 {
            tunnel: [w209 FALSE ("status")] -> w206
            tunnel: w202 -> [w208 _]
            frame False {
              n84 = Unbundle By Name(w208) -> ("status"=w209:bool)
              n85 = call <userlib>:"checkForError.vi"("Error In"=w208) -> ()  [unwired: 9 in, 2 out]
            }
            frame True {
            }
          }
          n86 = Or(x=w201, y=w205) -> (x .or. y?=w204:bool)
        }
        n87 = Enqueue Element(queue=w198, element=Host_State."Acquire", error in (no error)=w194) -> ()  [unwired: 1 in, 3 out]
        n88 = while "Dequeue elements in the PAS error queue" {
          tunnel: [w251] -> w196 mode=indexing
          stop <- w249 stop-if-true
          n89 = shared-variable "RT PXI Target\\PAS_Var.lvlib\\Error"(10 ("ms timeout (0)")) -> (w247:errorcluster, error out=w248:errorcluster, w246:bool)  [unwired: 1 in, 1 out]
          n90 = Unbundle By Name(w248) -> ("status"=w250:bool)
          n91 = case shown="False" w246 {
            tunnel: [w254 FALSE ("status")] -> w251
            tunnel: w247 -> [w253 _]
            frame False {
              n92 = Unbundle By Name(w253) -> ("status"=w254:bool)
              n93 = call <userlib>:"checkForError.vi"("Error In"=w253) -> ()  [unwired: 9 in, 2 out]
            }
            frame True {
            }
          }
          n94 = Or(x=w246, y=w250) -> (x .or. y?=w249:bool)
        }
        n95 = Or Array Elements(Boolean array=w182) -> (logical OR=w181:bool)
        n96 = case shown="True" w181 {
          selector: w181 -> [_ w200]
          frame False {
          }
          frame True {
            "genError" <- w200
          }
        }
        n97 = Or Array Elements(Boolean array=w196) -> (logical OR=w184:bool)
        n98 = case shown="True" w184 {
          selector: w184 -> [_ w211]
          frame False {
          }
          frame True {
            "pasErr" <- w211
          }
        }
        n99 = Current VI's Menubar() -> (w186:refnum<k9>)
        n100 = Get Menu Item Info(7:"sv::CLAP Data" ("item tag"), 11:w186) -> (1:w187:bool)  [unwired: 1 in, 6 out]
        n101 = case "Write CLAP Data" shown="True" w187 {
          tunnel: [w213 w218] -> w190
          tunnel: w189 -> [w213 w221]
          tunnel: [_ w214] -> w183
          frame False {
          }
          frame True {
            n102 = call "File Status.vi"("Data Path"=path "C:/CRD_PAS Data/CLAP", "ext"=".txt", "fileRefIn"=w221) -> ("error out"=w215:errorcluster, "fileRefOut"=w220:refnum<file>)  [unwired: 7 in]
            n103 = shared-variable "RT PXI Target\\General.lvlib\\CLAP Data"(error in=w215) -> (w217:string, error out=w216:errorcluster, w219:bool)  [unwired: 1 in]
            n104 = case shown="False" w219 {
              tunnel: w220 -> [w227 w235]
              tunnel: [w233 w235] -> w218
              tunnel: w217 -> [w229 _]
              tunnel: w216 -> [w228 w234]
              tunnel: [w224 w234] -> w214
              frame False {
                n105 = Format Date/Time String(time format string (%c)="%Y%m%dT%H:%M:%SZ,", UTC format=TRUE ("want seconds? (F)")) -> (date/time string=w230:string)  [unwired: 1 in]
                n106 = Concatenate Strings(w230, w229, "\r\n") -> (w225:string)
                n107 = Write to Text File(file (use dialog)=w227, text=w225, error in=w228) -> (refnum out=w233:refnum<file>, error out=w224:errorcluster)  [unwired: 1 in, 1 out]
              }
              frame True {
              }
            }
          }
        }
        n108 = while "Dequeue elements in CRDS error queue" {
          tunnel: [w238] -> w193 mode=indexing
          stop <- w239 stop-if-true
          n109 = shared-variable "RT PXI Target\\CRDS_Server.lvlib\\error"(10 ("ms timeout (0)")) -> (w237:errorcluster, error out=w242:errorcluster, w236:bool)  [unwired: 1 in, 1 out]
          n110 = case shown="False" w236 {
            tunnel: [w244 FALSE ("status")] -> w238
            tunnel: w237 -> [w243 _]
            frame False {
              n111 = Unbundle By Name(w243) -> ("status"=w244:bool)
              n112 = call <userlib>:"checkForError.vi"("Error In"=w243) -> ()  [unwired: 9 in, 2 out]
            }
            frame True {
            }
          }
          n113 = Unbundle By Name(w242) -> ("status"=w241:bool)
          n114 = Or(x=w236, y=w241) -> (x .or. y?=w239:bool)
        }
        n115 = Or Array Elements(Boolean array=w193) -> (logical OR=w185:bool)
        n116 = case shown="True" w185 {
          selector: w185 -> [_ w212]
          frame False {
          }
          frame True {
            "crdError" <- w212
          }
        }
      }
      frame "Write PAS Data" {
        # "Update all UI elements - update waveforms as indicated by the user."
        # "If the UI is just coming up or if the speaker is active, log the current resonant frequency and time of calibration."
        n117 = Current VI's Menubar() -> (w284:refnum<k9>)
        n118 = Get Menu Item Info(7:"Save" ("item tag"), 8:w278, 11:w284) -> (0:w282:errorcluster, 4:w281:bool)  [unwired: 5 out]
        n119 = case shown="True" w281 {
          tunnel: w282 -> [w296 w304]
          tunnel: w269 -> [w297 w299]
          tunnel: [w297 w301] -> w275
          tunnel: [w296 w300] -> w270
          tunnel: w266 -> [_ w303]
          frame False {
          }
          frame True {
            n120 = call-dynamic "Write Coded Binary.vi"("error in"=w304, "filter"=w303, "PAS Data in"=w299) -> ("error out"=w302:errorcluster, "PAS Data out"=w298:refnum<class "cPAS Data.lvclass">)  [unwired: 7 in]
            n121 = call "Write Remaining Data.vi"("error in"=w302, "cPAS Data in"=w298) -> ("error out"=w300:errorcluster, "cPAS Data out"=w301:refnum<class "cPAS Data.lvclass">)  [unwired: 8 in]
          }
        }
        n122 = property class="cPAS Data"(reference=w275, error in=w270) -> (error out=w272:errorcluster, "Drive"=w260:bool, "Time"=w259:timestamp, "Serial Data"=w274:refnum<class "Data.lvclass">[], "Cell Data"=w273:refnum<class "PAS Cell Data.lvclass">[], "Thum"=w268:cluster{"Hum 1":sgl, "Hum 2":sgl}, "dcVolts"=→"dcVolts":T27)  [unwired: 1 out]
        "pasSpk" <- w260
        "pasTime" <- w259
        n123 = Unbundle By Name(w268) -> ("Hum 1"=w267:sgl)
        "Thum" <- w267
        n124 = call "Sort Serial Data.vi"("error in"=w272, "SerialData"=w274) -> ("error out"=w271:errorcluster, "acatDataOut"=w289:T28, "TEC Data"=→"tecP":T29, 3:→"pasTte")  [unwired: 6 in]
        "pasACat" <- w289
        n125 = Cluster To Array(cluster=w289) -> (array=w292:cluster{"Q":sgl, "T":sgl, "P":sgl}[])
        n126 = To Long Integer(number="cell") -> (32bit integer=w261:i32)
        n127 = for {
          tunnel: w273 -> [w309] mode=indexing
          tunnel: [w338] -> w294 mode=indexing
          tunnel: [w339] -> w295 mode=indexing
          tunnel: [w325] -> w293 mode=indexing
          tunnel: w271 -> [w312]
          tunnel: w292 -> [w335] mode=indexing
          tunnel: [w336] -> w285 mode=indexing
          tunnel: w261 -> [w315]
          tunnel: [w307] -> w287 mode=indexing
          tunnel: [w316] -> w280 mode=indexing
          tunnel: w267 -> [w321]
          tunnel: [w306] -> w258 mode=indexing
          i -> [w323]
          n128 = To More Specific Class(target class=refnum<class "cPAS Cell Data.lvclass"> refnum ("cPAS Cell"), reference=w309, error in=w312) -> (specific class reference=w308:refnum<class "cPAS Cell Data.lvclass">, error out=w311:errorcluster)
          n129 = Cluster To Array(cluster=w335) -> (array=w333:sgl[])
          n130 = Equal?(x=w315, y=w323) -> (x = y?=w342:bool)
          n131 = Equal To 0?(x=w323) -> (x = 0?=w322:bool)
          n132 = call "Read derived.vi"("error in"=w311, "PAS Cell Data in"=w308) -> ("error out"=w341:errorcluster, "derived"=w318:T30, "PAS Cell Data out"=w332:refnum<class "cPAS Cell Data.lvclass">)  [unwired: 7 in]
          n133 = To Single Precision Float(number=w318) -> (single precision float=w317:T31)
          n134 = Unbundle(w317) -> ("f0"=w325:sgl, "IA"=w331:sgl, "Q"=w324:sgl, "max"=w326:sgl[], "deltaPhi"=w330:sgl, "tau"=w329:sgl, "noiseLim"=w328:sgl, "ext"=w327:sgl)
          n135 = Select(t=w321, s=w322, f=sgl nan) -> (s? t:f=w319:sgl)
          n136 = Build Array (concatenate)(w325, w331, w324, w326, w330, w329, w328, w327) -> (w316:sgl[])
          n137 = case shown="True" w342 {
            tunnel: w332 -> [w344 w352]
            tunnel: w341 -> [w343 w345]
            tunnel: w325 -> [_ w361]
            tunnel: w324 -> [_ w360]
            tunnel: [w344 w347] -> w314
            tunnel: [w343 w346] -> w305
            frame False {
            }
            frame True {
              w358 = 1.0
              n138 = property class="cPAS Cell"(reference=w352, error in=w345) -> (reference out=w347:refnum<class "cPAS Cell Data.lvclass">, error out=w346:errorcluster, "Mic Time"=→"micTime":waveform(i16), "Photodiode"=→"diodeTime":waveform(i16), "Fitted Data"=w349:waveform(sgl), "Mic Frequency"=w348:waveform(sgl))
              n139 = Unbundle By Name(w349) -> ("Y"=w359:sgl[])
              n140 = Unbundle By Name(w348) -> ("Y"=w362:sgl[])
              n141 = Bundle(500, w358, "Y"=w362) -> (w355:cluster{i32, dbl, "Y":sgl[]})  [unwired: 1 in]
              n142 = Bundle(0, w358, "Y"=w359) -> (w356:cluster{i32, dbl, "Y":sgl[]})  [unwired: 1 in]
              n143 = Build Array(w356, w355) -> (→"micFreq":cluster{i32, dbl, "Y":sgl[]}[])
              "f0" <- w361
              "Q" <- w360
            }
          }
          n144 = property class="cPAS Cell"(reference=w314, error in=w305) -> (error out=w307:errorcluster, "Housekeeping"=w313:T32, "Data Access:T2"=w306:sgl)  [unwired: 1 out]
          n145 = Unbundle By Name(w313) -> ("T"=w338:sgl, "RH"=w337:sgl, "TRH"=w340:sgl)
          n146 = Cluster To Array(cluster=w313) -> (array=w334:sgl[])
          n147 = Build Array (concatenate)(w333, w334, w319, w306) -> (w336:sgl[])
          n148 = Bundle("RH"=w337, "TRH"=w340) -> (w339:cluster{"RH":sgl, "TRH":sgl})  [unwired: 1 in]
        }
        n149 = case shown="True" w260 {
          tunnel: w293 -> [_ _]
          tunnel: w259 -> [_ w363]
          frame False {
          }
          frame True {
            "lastCal" <- w363
          }
        }
        n150 = Bundle(w280, "Time"=w259) -> (w263:cluster{sgl[][], "Time":timestamp})  [unwired: 1 in]
        "pasDerData" <- w263
        n151 = Array To Cluster(array=w294) -> (cluster=→"PASCellT":T11)
        n152 = Bundle(cluster=w263, w285) -> (→"pasHK":cluster{sgl[][], "Time":timestamp})  [unwired: 1 in]
        n153 = Array To Cluster(array=w258) -> (cluster=→"PASCellT2":T11)
        n154 = Array To Cluster(array=w295) -> (cluster=→"pasRH":T33)
        n155 = Merge Errors(w287) -> (w279:errorcluster)
      }
      frame "Write CRD Data" {
        n156 = Current VI's Menubar() -> (w385:refnum<k9>)
        n157 = Get Menu Item Info(7:"Save" ("item tag"), 8:w382, 11:w385) -> (0:w381:errorcluster, 4:w383:bool)  [unwired: 5 out]
        n158 = case shown="True" w383 {
          tunnel: w365 -> [w409 w414]
          tunnel: [w409 w413] -> w364
          tunnel: w381 -> [w408 w412]
          tunnel: [w408 w411] -> w380
          tunnel: w372 -> [_ w410]
          frame False {
          }
          frame True {
            n159 = call-dynamic "Write Class Data to File.vi"("error in"=w412, "filter"=w410, "cCRDS Data in"=w414) -> ("error out"=w411:errorcluster, "cCRDS Data out"=w413:refnum<class "cCRDS Data.lvclass">)  [unwired: 6 in, 1 out]
          }
        }
        n160 = property class="cCRDS Data" props=["Alicat Data", "Data Access:Cell Data", "Humidifier T", "Time", "Pressure", "vData", "Alicat Data"](reference=w364, error in=w380) -> (error out=w379:errorcluster, "Data Access:Cell Data"=w377:refnum<class "CRDS Cell Data.lvclass">[], "Humidifier T"=w368:cluster{"Hum 1":sgl, "Hum 2":sgl}, "Time"=w367:timestamp, "Pressure"=w392:sgl[], "vData"=w390:cluster{"TRH":dbl, "RH":dbl}[], "Alicat Data"=w366:T34)  [unwired: 2 out]
        "TRHin" <- w368
        "crdTime" <- w367
        n161 = local read "crd::rhctl"() -> (w371:bool)
        n162 = case shown="True" w371 {
          frame False {
          }
          frame True {
            n163 = shared-variable "RT PXI Target\\CRDS_Server.lvlib\\Tsp"() -> (w407:sgl[])  [unwired: 1 in, 1 out]
            n164 = Array To Cluster(array=w407) -> (cluster=w406:T35)
            n165 = local write "crd::tec::T"(w406) -> ()
          }
        }
        n166 = Array To Cluster(array=w392) -> (cluster=→"P":T36)
        n167 = Array To Cluster(array=w390) -> (cluster=→"vaisalaData":T37)
        n168 = Cluster To Array(cluster=w368) -> (array=w370:sgl[])
        n169 = for {
          tunnel: w377 -> [w431] mode=indexing
          tunnel: [w430] -> w402 mode=indexing
          tunnel: [w428] -> w401 mode=indexing
          tunnel: [w421] -> w387 mode=indexing
          tunnel: w379 -> [w427]
          tunnel: [w425] -> w378 mode=indexing
          tunnel: w370 -> [w420]
          i -> [w424]
          n170 = property class="CRDS Cell"(reference=w431, error in=w427) -> (error out=w425:errorcluster, "Data Access:Ringdowns"=w430:i16[][], "Data Access:extParam"=w429:T38, "Data Access:Housekeeping"=w426:T39)  [unwired: 1 out]
          n171 = case shown="7" w424 {
            tunnel: [sgl nan w434 w437] -> w422
            tunnel: w420 -> [_ w435 w438]
            frame 0, Default {
            }
            frame 6 {
              n172 = Index Array(array=w435, index=0) -> (element=w434:sgl)
            }
            frame 7 {
              n173 = Index Array(array=w438, index=1) -> (element=w437:sgl)
            }
          }
          n174 = Cluster To Array(cluster=w429) -> (array=w428:sgl[])
          n175 = Cluster To Array(cluster=w426) -> (array=w423:sgl[])
          n176 = Build Array (concatenate)(w423, w422) -> (w421:sgl[])
        }
        "Ringdown" <- w402
        n177 = Split 1D Array(array=w366, index=1) -> (first subarray=w399:T34, second subarray=w400:T34)
        n178 = Bundle(w387, "Time"=w367) -> (→"crdHK":cluster{sgl[][], "Time":timestamp})  [unwired: 1 in]
        n179 = Merge Errors(w378) -> (w373:errorcluster)
        n180 = for {
          tunnel: w400 -> [w419] mode=indexing
          tunnel: [w418] -> w398 mode=indexing
          n181 = Unbundle By Name(w419) -> ("Q"=w417:sgl, "T"=w416:sgl, "P"=w415:sgl)
          n182 = Bundle("Q"=w417, "T"=w416, "P"=w415) -> (w418:cluster{"Q":sgl, "T":sgl, "P":sgl})  [unwired: 1 in]
        }
        n183 = Bundle("Data Access:extParam"=w401, "Time"=w367) -> (→"extWvfm":T40)  [unwired: 1 in]
        n184 = Index Array(array=w399) -> (element=w394:T41)  [unwired: 1 in]
        n185 = Unbundle By Name(w394) -> ("Q"=w376:sgl, "T"=w375:sgl, "P"=w374:sgl)
        n186 = Bundle("Q"=w376, "T"=w375, "P"=w374) -> (w397:cluster{"Q":sgl, "T":sgl, "P":sgl})  [unwired: 1 in]
        n187 = Build Array (concatenate)(w398, w397) -> (w396:cluster{"Q":sgl, "T":sgl, "P":sgl}[])
        n188 = Array To Cluster(array=w396) -> (cluster=→"alctData":T28)
        n189 = disable-structure shown="Disabled" {
          frame Disabled {
            n190 = property on="Ringdown" class="Ringdown (strict)"() -> ("Property"=→"rdError":bool)  [unwired: 2 in, 2 out]
          }
          frame Enabled {
          }
        }
      }
      frame "Quit" {
        w458 = FALSE ("checked")
        w465 = FALSE ("manSpk")
        n191 = Release Queue(queue=w470, error in (no error)=w469) -> (error out=w442:errorcluster)  [unwired: 1 in, 2 out]
        n192 = Not A Number/Path/Refnum?(number/path/refnum=w443) -> (NaN/Path/Refnum?=w444:bool)
        n193 = case shown="False" w444 {
          tunnel: w443 -> [w473 _]
          tunnel: w442 -> [w472 w474]
          tunnel: [w471 w474] -> w441
          frame False {
            n194 = Close File(refnum=w473, error in=w472) -> (error out=w471:errorcluster)  [unwired: 1 out]
          }
          frame True {
          }
        }
        n195 = call <userlib>:"destructor_error_logger.vi"("error in (no error)"=w441) -> ("error out"=w457:errorcluster)  [unwired: 10 in]
        n196 = Current VI's Menubar() -> (w463:refnum<k9>)
        n197 = Set Menu Item Info(6:w458, 7:"Save" ("item tag"), 8:w457, 11:w463) -> (0:w461:errorcluster, 3:w460:refnum<k9>)  [unwired: 3 in]
        n198 = Two Button Dialog(message="Shutdown server?", 1:"Cancel" ("F button name (\"Cancel\")"), 2:"Shutdown" ("T button name (\"OK\")")) -> (T button?=w448:bool)
        n199 = Set Menu Item Info(6:w458, 7:"autoSpk" ("item tag"), 8:w461, 11:w460) -> (0:w440:errorcluster)  [unwired: 3 in, 1 out]
        n200 = property on="Write" class="Bool (strict)"(error in=w440, "Value"=w465, "Blinking"=w465) -> (error out=w464:errorcluster)  [unwired: 1 in, 1 out]
        n201 = case shown="True" w448 {
          tunnel: w464 -> [w475 w479]
          tunnel: [w475 w480] -> w456
          frame False {
          }
          frame True {
            w477 = FALSE ("manSpk")
            n202 = shared-variable "RT PXI Target\\PAS_Var.lvlib\\manSpk"(w477, error in=w479) -> (error out=w478:errorcluster)
            n203 = shared-variable "RT PXI Target\\General.lvlib\\stop"(TRUE, error in=w478) -> (error out=w481:errorcluster)
            n204 = shared-variable "RT PXI Target\\General.lvlib\\O3cal"(w477, error in=w481) -> (error out=w480:errorcluster)
          }
        }
        n205 = Unbundle By Name(w456) -> ("code"=w468:i32)
        n206 = Equal?(x=w468, y=-1950679035) -> (x = y?=w466:bool)
        n207 = case shown="True" w466 {
          tunnel: w456 -> [w482 _]
          tunnel: [w482 errorcluster {"status"=FALSE, "code"=0, "source"=""} ("error IO")] -> w454
          frame False {
          }
          frame True {
          }
        }
        n208 = call "Display and Save Single Shot Taus.vi"("error in"=w454, "state"=tau_state."Close") -> ("error out"=w453:errorcluster)  [unwired: 9 in]
      }
    }
    n209 = call <userlib>:"checkForError.vi"("Error In"=w18) -> ("error out"=w17:errorcluster)  [unwired: 9 in, 1 out]
  }
  n210 = while "Listen for user generated events" {
    tunnel: w2 -> [w488]
    i -> [w486]
    stop <- w489 stop-if-true
    n211 = Equal To 0?(x=w486) -> (x = 0?=w485:bool)
    n212 = case shown="True" w485 {
      tunnel: [-1 0] -> w487
      frame False {
      }
      frame True {
      }
    }
    n213 = event shown="[11] \"swDispl\": Value Change" {
      selector: _ -> [_ _ _ _ _ _ _ _ _ _ _ _]
      dyn-events: _ -> [_ _ _ _ _ _ _ _ _ _ _ _]
      timeout: w487 -> [_ _ _ _ _ _ _ _ _ _ _ _]
      tunnel: [FALSE ("Discard?") _ _ _ w549 _ w567 _ _ _ _ FALSE ("Discard?")] -> w489
      tunnel: w488 -> [_ _ _ _ w552 _ w566 _ _ _ _ _]
      tunnel: [w492 w542 w543 w546 w550 w559 w568 w734 w748 w761 w767 _] -> w484
      event Timeout {
        w495 = TRUE ("Clear Graph")
        w500 = T43 [{"Name"="RH", "Line Width"=2, "Line Style"=0, "Color"=1985280}, {"Name"="Dry", "Line Width"=2, "Line Style"=1, "Color"=1985280}, {"Name"="Dry", "Line Width"=2, "Line Style"=0, "Color"=16711680}, {"Name"="Dry", "Line Width"=2, "Line Style"=0, "Color"=16860}, {"Name"="Denuded", "Line Width"=2, "Line Style"=1, "Color"=16860}] ("Plot Details")
        w520 = T43 [{"Name"="Denuded", "Line Width"=2, "Line Style"=0, "Color"=16711680}, {"Name"="Denuded", "Line Width"=2, "Line Style"=1, "Color"=16860}, {"Name"="Gas", "Line Width"=2, "Line Style"=0, "Color"=33023}, {"Name"="Dry", "Line Width"=2, "Line Style"=0, "Color"=16512}, {"Name"="Dry", "Line Width"=2, "Line Style"=0, "Color"=8388672}, {"Name"="Dry", "Line Width"=2, "Line Style"=1, "Color"=6618880}, {"Name"="Med RH", "Line Width"=2, "Line Style"=1, "Color"=1985280}, {"Name"="High RH", "Line Width"=2, "Line Style"=1, "Color"=32832}] ("Plot Details")
        # "Initialize interface stuff; system times out only the first time."
        n214 = event-data() -> ()  [unwired: 1 in, 1 out]
        n215 = Cluster To Array(cluster="swDispl") -> (array=w505:bool[])
        n216 = local write "pasTECEn"(T42 {"c 1"=TRUE, "c 2"=TRUE, "c 3"=TRUE, "c 4"=TRUE, "c 5"=TRUE} ("pasTECEn")) -> ()
        n217 = Array Size(array=w505) -> (size(s)=w506:i32)
        n218 = local write "tabCtl"(T2."main" ("tabCtl")) -> ()
        n219 = local write "pasErr"(TRUE ("Value")) -> ()
        n220 = Initialize Array(FALSE, w506) -> (w501:bool[])
        n221 = Replace Array Subset(array=w501, new element=TRUE ("new element/subarray")) -> (w507:bool[])  [unwired: 1 in]
        n222 = for {
          N: 8 -> [_]
          tunnel: "Channel " -> [w525]
          tunnel: [w524] -> w517 mode=indexing
          i -> [w527]
          n223 = Increment(x=w527) -> (x+1=w526:i32)
          n224 = Format Into String(initial string=w525, w526) -> (resulting string=w524:string)  [unwired: 2 in, 1 out]
        }
        n225 = Array To Cluster(array=w507) -> (cluster=w504:T44)
        n226 = local write "swDispl"(w504) -> ()
        n227 = Array Subset(array=w517, length=5) -> (w498:string[])  [unwired: 1 in]
        n228 = property on="extWvfm" class="2D Buffer Display (strict)"("Y Axis Labels"=string[] ["tau (us)", "Corrected tau0 (us)", "Extinction (Mm-1)", "Corrected Extinction (Mm-1)", "Std. Dev. in tau (us)", "Error in tau", "Corrected tau (us)", "tau0 (us)", "Max Amplitude"], "Channels"=w517, "Variables"=string[] ["Tau", "Corr.  tau0", "Extinction", "Corrected Extinction", "Std. Dev. in tau", "Error in tau", "Corrected tau", "tau0", "Max Amplitude"], "Plot Details"=w520, "Clear Graph"=w495) -> (error out=w513:errorcluster)  [unwired: 2 in, 1 out]
        n229 = property on="crdHK" class="2D Buffer Display (strict)"(error in=w513, "Y Axis Labels"=string[] ["fRH", "Flow Rate (lpm)", "Tmean (degC)", "fext", "Relative Humidity (%)", "Pressure (mb)", "Temperature (degC)", "Saturator Temperature (degC)"], "Channels"=w517, "Variables"=string[] ["fRH", "Flow Rate", "Tmean", "fext", "Relative Humidity", "Pressure", "Temperature", "Saturator Temperature"], "Plot Details"=w520, "Clear Graph"=w495) -> (error out=w516:errorcluster)  [unwired: 1 in, 1 out]
        n230 = property on="pasHK" class="2D Buffer Display (strict)"(error in=w516, "Y Axis Labels"=string[] ["Flow Rate (lpm)", "MFC Temperature (lpm)", "Pressure (mb)", "TEC Thermistor Temperature (degC)", "Vaisala Temperature (degC)", "Relative Humidity (%)", "Laser RMS", "Saturator Temperature (degC)", "Thermistor "], "Plot Details"=w500, "Variables"=string[] ["Flow Rate", "MFC Temperature", "Pressure", "TEC Thermistor Temperature", "Vaisala Temperature", "Relative Humidity", "Laser RMS", "Saturator Temperature", "Thermistor Temperature"], "Channels"=w498, "Clear Graph"=w495) -> (error out=w499:errorcluster)  [unwired: 1 in, 1 out]
        n231 = property on="pasDerData" class="2D Buffer Display (strict)"(error in=w499, "Y Axis Labels"=string[] ["f0 (Hz)", "Integrated Area", "Q", "Max Value", "Max Location (Hz)", "delta Phi", "tau", "Noise Limit", "Absorbtion (Mm^-1)"], "Plot Details"=w500, "Variables"=string[] ["f0", "Integrated Area", "Q", "Max Value", "Max Location", "deltaPhi", "tau", "Noise Limit", "Absorbtion"], "Channels"=w498, "Clear Graph"=w495) -> (error out=w492:errorcluster)  [unwired: 1 in, 1 out]
      }
      event "crd::rhctl": Value Change {
        w535 = T23."Disabled and Grayed Out" ("Disabled")
        w534 = T23."Enabled" ("Disabled")
        # "If there is no flow, on the humidified channels, then the user can not control based on RH."
        n232 = event-data() -> ("NewVal"=w530:bool)  [unwired: 1 in]
        n233 = local read "crdFlows"() -> (w541:T7)
        n234 = Unbundle(w541) -> ("mRH"=w540:sgl, "hRH"=w539:sgl)  [unwired: 3 out]
        n235 = Equal To 0?(x=w540) -> (x = 0?=w538:bool)
        n236 = Equal To 0?(x=w539) -> (x = 0?=w537:bool)
        n237 = Or(x=w538, y=w537) -> (x .or. y?=w531:bool)
        n238 = Select(t=FALSE, s=w531, f=w530) -> (s? t:f=w528:bool)
        n239 = local write "crd::rhctl"(w528) -> ()
        n240 = Select(t=w534, s=w528, f=w535) -> (s? t:f=w536:T23)
        n241 = property on="crd::rh" class="Clust (strict)"("DisabledEnum"=w536) -> (error out=w532:errorcluster)  [unwired: 2 in, 1 out]
        n242 = Select(t=w535, s=w528, f=w534) -> (s? t:f=w533:T23)
        n243 = property on="crd::tec::T" class="Clust (strict)"(error in=w532, "DisabledEnum"=w533) -> (error out=w542:errorcluster)  [unwired: 1 in, 1 out]
      }
      event "crd::tec::T": Value Change {
        n244 = event-data() -> ("NewVal"=w545:cluster{"hum":sgl, "dry":sgl})  [unwired: 1 in]
        n245 = Cluster To Array(cluster=w545) -> (array=w544:sgl[])
        n246 = shared-variable "RT PXI Target\\CRDS_Server.lvlib\\Tsp"(w544) -> (error out=w543:errorcluster)  [unwired: 1 in]
      }
      event "crd::rh": Value Change {
        n247 = event-data() -> ("NewVal"=w548:cluster{"hum":sgl, "dry":sgl})  [unwired: 1 in]
        n248 = Cluster To Array(cluster=w548) -> (array=w547:sgl[])
        n249 = shared-variable "RT PXI Target\\CRDS_Server.lvlib\\RHsp"(w547) -> (error out=w546:errorcluster)  [unwired: 1 in]
      }
      event Panel Close? {
        w549 = TRUE ("Discard?")
        # "Send the message to stop the session; the server will close the connection and the host should close gracefully as the display loop realizes the connections is closed."
        n250 = event-data() -> ()  [unwired: 1 in, 1 out]
        n251 = Enqueue Element(queue=w552, element=Host_State."Quit") -> (error out=w550:errorcluster)  [unwired: 2 in, 2 out]
        n252 = event-data("Discard?"=w549) -> ()  [unwired: 1 in, 1 out]
      }
      event "pas::rhctl": Value Change {
        w562 = T23."Disabled and Grayed Out" ("Disabled")
        w563 = T23."Enabled" ("Disabled")
        # "Do not allow the user to control saturator TEC temperature based on RH if there is no flow through the cell."
        n253 = event-data() -> ()  [unwired: 1 in, 1 out]
        n254 = local read "pasFlows"() -> (w558:T17)
        n255 = Unbundle By Name(w558) -> ("Cell 1"=w557:sgl)
        n256 = Equal To 0?(x=w557) -> (x = 0?=w556:bool)
        n257 = Select(t=FALSE, s=w556, f="pas::rhctl") -> (s? t:f=w553:bool)
        n258 = local write "pas::rhctl"(w553) -> ()
        n259 = Select(t=w562, s=w553, f=w563) -> (s? t:f=w561:T23)
        n260 = Select(t=w563, s=w553, f=w562) -> (s? t:f=w564:T23)
        n261 = property on="pas::satT" class="DigNum (strict)"("DisabledEnum"=w561) -> (error out=w560:errorcluster)  [unwired: 2 in, 1 out]
        n262 = property on="pas::rh" class="DigNum (strict)"(error in=w560, "DisabledEnum"=w564) -> (error out=w559:errorcluster)  [unwired: 1 in, 1 out]
      }
      event Menu Selection (User) {
        n263 = event-data() -> ("ItemTag"=w569:string, "MenuRef"=w565:refnum<k9>)  [unwired: 1 in]
        n264 = case shown="\"autoSpk\"" w569 {
          selector: w569 -> [w576 w599 w613 w629 w646 _ _ _ w676 _ w684 _ _ _ _ _ _ w703 _ _ _ _]
          tunnel: w565 -> [w580 w600 w616 w632 w648 _ _ _ w677 _ w682 _ _ _ _ _ _ w706 _ _ _ _]
          tunnel: [w571 w581 w602 w618 w633 w651 _ _ w670 _ w680 w689 _ _ _ w693 _ w700 w708 w710 w716 w718] -> w568
          tunnel: [FALSE FALSE _ FALSE FALSE FALSE FALSE FALSE FALSE FALSE FALSE FALSE FALSE FALSE FALSE TRUE w697 FALSE FALSE _ _ _] -> w567
          tunnel: w566 -> [_ _ _ _ _ _ _ _ _ _ _ _ _ _ _ w695 _ _ _ _ _ _]
          frame "Align" {
            # "Set the mode on the CRD to align."
            n265 = Get Menu Item Info(7:w576, 11:w580) -> (0:w577:errorcluster, 3:w578:refnum<k9>, 4:w572:bool)  [unwired: 1 in, 4 out]
            n266 = Not(x=w572) -> (.not. x?=w579:bool)
            n267 = Set Menu Item Info(6:w579, 7:w576, 8:w577, 11:w578) -> (0:w574:errorcluster, 3:w575:refnum<k9>)  [unwired: 3 in]
            n268 = Set Menu Item Info(6:w572, 7:"Sample" ("item tag"), 8:w574, 11:w575) -> (0:w571:errorcluster)  [unwired: 3 in, 1 out]
          }
          frame "autoFilt" {
            n269 = Get Menu Item Info(7:w599, 11:w600) -> (0:w597:errorcluster, 3:w598:refnum<k9>, 4:w596:bool)  [unwired: 1 in, 4 out]
            n270 = Not(x=w596) -> (.not. x?=w584:bool)
            n271 = Set Menu Item Info(6:w584, 7:w599, 8:w597, 11:w598) -> (0:w583:errorcluster)  [unwired: 3 in, 1 out]
            n272 = shared-variable "RT PXI Target\\General.lvlib\\flags"(error in=w583) -> (w590:u8, error out=w591:errorcluster)
            n273 = Number To Boolean Array(number=w590) -> (Boolean array=w589:bool[])
            n274 = Replace Array Subset(array=w589, new element=w584, index=3) -> (w587:bool[])
            n275 = Boolean Array To Number(Boolean array=w587) -> (number=w586:u32)
            n276 = Select(t=T23."Disabled and Grayed Out" ("Disabled"), s=w584, f=T23."Enabled") -> (s? t:f=w593:T23)
            n277 = To Unsigned Byte Integer(number=w586) -> (unsigned 8bit integer=w585:u8)
            n278 = shared-variable "RT PXI Target\\General.lvlib\\flags"(w585, error in=w591) -> (error out=w582:errorcluster)
            n279 = property on="filter" class="Bool (strict)"(error in=w582, "DisabledEnum"=w593) -> (error out=w592:errorcluster)  [unwired: 1 in, 1 out]
            n280 = property on="bypass" class="Bool (strict)"(error in=w592, "DisabledEnum"=w593) -> (error out=w581:errorcluster)  [unwired: 1 in, 1 out]
          }
          frame "lSpkFilt" {
            n281 = Get Menu Item Info(7:w613, 11:w616) -> (0:w612:errorcluster, 3:w615:refnum<k9>, 4:w614:bool)  [unwired: 1 in, 4 out]
            n282 = Not(x=w614) -> (.not. x?=w603:bool)
            n283 = Set Menu Item Info(6:w603, 7:w613, 8:w612, 11:w615) -> (0:w604:errorcluster)  [unwired: 3 in, 1 out]
            n284 = shared-variable "RT PXI Target\\General.lvlib\\flags"(error in=w604) -> (w610:u8, error out=w611:errorcluster)
            n285 = Number To Boolean Array(number=w610) -> (Boolean array=w609:bool[])
            n286 = Replace Array Subset(array=w609, new element=w603, index=1) -> (w607:bool[])
            n287 = Boolean Array To Number(Boolean array=w607) -> (number=w606:u32)
            n288 = To Unsigned Byte Integer(number=w606) -> (unsigned 8bit integer=w605:u8)
            n289 = shared-variable "RT PXI Target\\General.lvlib\\flags"(w605, error in=w611) -> (error out=w602:errorcluster)
          }
          frame "O3Cal" {
            n290 = Get Menu Item Info(7:w629, 11:w632) -> (0:w631:errorcluster, 3:w630:refnum<k9>, 4:w628:bool)  [unwired: 1 in, 4 out]
            n291 = Not(x=w628) -> (.not. x?=w619:bool)
            n292 = Set Menu Item Info(6:w619, 7:w629, 8:w631, 11:w630) -> (0:w620:errorcluster)  [unwired: 3 in, 1 out]
            n293 = shared-variable "RT PXI Target\\General.lvlib\\flags"(error in=w620) -> (w626:u8, error out=w627:errorcluster)
            n294 = Number To Boolean Array(number=w626) -> (Boolean array=w625:bool[])
            n295 = Replace Array Subset(array=w625, new element=w619, index=4) -> (w623:bool[])
            n296 = Boolean Array To Number(Boolean array=w623) -> (number=w622:u32)
            n297 = To Unsigned Byte Integer(number=w622) -> (unsigned 8bit integer=w621:u8)
            n298 = shared-variable "RT PXI Target\\General.lvlib\\flags"(w621, error in=w627) -> (error out=w618:errorcluster)
          }
          frame "autoSpk" {
            # "Override speaker duty cycle on PAS."
            n299 = Get Menu Item Info(7:w646, 11:w648) -> (0:w644:errorcluster, 3:w647:refnum<k9>, 4:w645:bool)  [unwired: 1 in, 4 out]
            n300 = Not(x=w645) -> (.not. x?=w638:bool)
            n301 = Set Menu Item Info(6:w638, 7:w646, 8:w644, 11:w647) -> (0:w634:errorcluster)  [unwired: 3 in, 1 out]
            n302 = shared-variable "RT PXI Target\\General.lvlib\\flags"(error in=w634) -> (w641:u8, error out=w642:errorcluster)
            n303 = Number To Boolean Array(number=w641) -> (Boolean array=w640:bool[])
            n304 = Replace Array Subset(array=w640, new element=w638, index=0) -> (w637:bool[])
            n305 = Boolean Array To Number(Boolean array=w637) -> (number=w636:u32)
            n306 = To Unsigned Byte Integer(number=w636) -> (unsigned 8bit integer=w635:u8)
            n307 = shared-variable "RT PXI Target\\General.lvlib\\flags"(w635, error in=w642) -> (error out=w633:errorcluster)
          }
          frame "how" {
            # "Open the help file - location will differ depending on what the type of application is."
            n308 = property class="App"() -> (error out=w649:errorcluster, "App.Kind"=w655:T22)  [unwired: 2 in, 1 out]
            n309 = Current VI's Path() -> (path=w660:path)
            n310 = Strip Path(path=w660) -> (stripped path=w654:path)  [unwired: 1 out]
            n311 = case shown="\"Run Time System\"" w655 {
              tunnel: w654 -> [w662 w667]
              tunnel: [w662 w664] -> w653
              tunnel: ["Help" ("name or relative path") "Support" ("name or relative path")] -> w652
              frame "Development System", Default {
              }
              frame "Run Time System" {
                n312 = Strip Path(path=w667) -> (stripped path=w666:path)  [unwired: 1 out]
                n313 = Strip Path(path=w666) -> (stripped path=w665:path)  [unwired: 1 out]
                n314 = Strip Path(path=w665) -> (stripped path=w664:path)  [unwired: 1 out]
              }
            }
            n315 = Build Path(base path=w653, name or relative path=w652) -> (appended path=w656:path)
            n316 = Build Path(base path=w656, name or relative path="CRDS_PAS Help.chm") -> (appended path=w658:path)
            n317 = Control Online Help(1:w649, 2:w658, 4:enum16{"Contents", "Key", "Close"}."Contents" ("Operation")) -> (0:w651:errorcluster)  [unwired: 1 in]
          }
          frame "notes" {
          }
          frame "cfg" {
          }
          frame "svRD" {
            n318 = Get Menu Item Info(7:w676, 11:w677) -> (0:w674:errorcluster, 3:w673:refnum<k9>, 4:w675:bool)  [unwired: 1 in, 4 out]
            n319 = Not(x=w675) -> (.not. x?=w671:bool)
            "svRDs" <- w671
            n320 = Set Menu Item Info(6:w671, 7:w676, 8:w674, 11:w673) -> (0:w670:errorcluster)  [unwired: 3 in, 1 out]
          }
          frame "restartCRDAI" {
          }
          frame "Sample" {
            # "Set the mode on the CRD to sample"
            n321 = Set Menu Item Info(6:TRUE ("checked"), 7:w684, 11:w682) -> (0:w686:errorcluster, 3:w687:refnum<k9>)  [unwired: 4 in]
            n322 = Set Menu Item Info(6:FALSE ("checked"), 7:"Align" ("item tag"), 8:w686, 11:w687) -> (0:w680:errorcluster)  [unwired: 3 in, 1 out]
          }
          frame "eLog" {
            n323 = call <userlib>:"openErrorLogWindow.vi"() -> ("error out"=w689:errorcluster)  [unwired: 11 in]
          }
          frame "NULL", Default {
            # "The default case for selections not implemented.  Does nothing."
          }
          frame "centCurs" {
            # "Center the cursors so that they can be repositioned.  This will not work if the PAS is not present."
          }
          frame "dTable" {
            # "Show the table containing the averages of the values recorded by the PAS and CRDS.  Values not returned correctly if the PAS is not connected."
          }
          frame "Exit" {
            n324 = Enqueue Element(queue=w695, element=Host_State."Quit") -> (error out=w693:errorcluster)  [unwired: 2 in, 2 out]
          }
          frame "cError" {
            w697 = FALSE
            # "Clear errors thrown on the PAS and CRDS"
            n325 = local write "pasErr"(w697) -> ()
            n326 = local write "crdError"(w697) -> ()
            n327 = local write "genError"(w697) -> ()
          }
          frame "Save" {
            # "Toggle the Save menu selection.  If writing, set the indicators to blink."
            n328 = Get Menu Item Info(7:w703, 11:w706) -> (0:w701:errorcluster, 3:w704:refnum<k9>, 4:w705:bool)  [unwired: 1 in, 4 out]
            n329 = Not(x=w705) -> (.not. x?=w702:bool)
            n330 = Set Menu Item Info(6:w702, 7:w703, 8:w701, 11:w704) -> (0:w698:errorcluster)  [unwired: 3 in, 1 out]
            n331 = property on="write" class="Bool (strict)"(error in=w698, "Value"=w702, "Blinking"=w702) -> (error out=w700:errorcluster)  [unwired: 1 in, 1 out]
          }
          frame "reboot" {
            n332 = call-poly <vilib>:"RT Restart Target.vi"("target address"="10.172.240.107") -> ("error out"=w708:errorcluster)  [unwired: 8 in, 2 out]
          }
          frame "eject" {
            n333 = shared-variable "RT PXI Target\\General.lvlib\\Ustatus"() -> (w715:bool[], error out=w711:errorcluster)  [unwired: 1 in]
            n334 = Replace Array Subset(array=w715, new element=TRUE ("new element/subarray"), index=1) -> (w712:bool[])
            n335 = shared-variable "RT PXI Target\\General.lvlib\\Ustatus"(w712, error in=w711) -> (error out=w710:errorcluster)
          }
          frame "sync" {
            n336 = Get Date/Time In Seconds() -> (seconds since 1Jan1904=w717:timestamp)
            n337 = shared-variable "RT PXI Target\\General.lvlib\\host_time"(w717) -> (error out=w716:errorcluster)  [unwired: 1 in]
          }
          frame "About" {
            n338 = Open VI Reference(vi path=path "C:/Users/mrichardson/Documents/Version Controlled LV Sw/PAS_CRDS new/About Screen.vi") -> (vi reference=w725:refnum<vi>, error out=w724:errorcluster)  [unwired: 5 in]
            n339 = invoke class="VI" method="Run VI"(reference=w725, error in=w724, "Wait until done"=FALSE ("Wait Until Done"), "Auto Dispose Ref"=TRUE ("Auto Dispose Reference")) -> (reference out=w721:refnum<vi>, error out=w720:errorcluster)  [unwired: 1 in, 3 out]
            n340 = property class="VI"(reference=w721, error in=w720, "Front Panel.Open"=TRUE ("Front Panel Window:Open")) -> (error out=w718:errorcluster)  [unwired: 1 out]
          }
        }
      }
      event "Qclap", "crdFlows", "QO3": Value Change {
        # "Do not allow the user to turn on CRD flows if there is no purge flow."
        n341 = event-data() -> ()  [unwired: 1 in, 1 out]
        n342 = local read "alctData"() -> (w732:T5)
        n343 = Unbundle By Name(w732) -> ("purge.Q"=w728:sgl)
        n344 = Less Or Equal?(x=w728, y=sgl 0.05) -> (x <= y?=w731:bool)
        n345 = case shown="True" w731 {
          tunnel: "crdFlows" -> [w744 w747]
          tunnel: [w744 w745] -> w729
          frame False {
          }
          frame True {
            w746 = sgl 0.0 ("denude")
            n346 = Bundle(cluster=w747, "denude"=w746, "dry"=w746, "mRH"=w746, "hRH"=w746) -> (w745:T7)  [unwired: 1 in]
            n347 = local write "crdFlows"(w745) -> ()
          }
        }
        n348 = Cluster To Array(cluster="pasFlows") -> (array=w737:sgl[])
        n349 = Unbundle(w729) -> ("denude"=w741:sgl, "dry"=w740:sgl, "mRH"=w739:sgl, "hRH"=w738:sgl, "purge"=w742:sgl)
        n350 = Build Array (concatenate)(w742, w741, w740, w739, w738, w737, "Qclap", "QO3") -> (w736:sgl[])
        n351 = shared-variable "RT PXI Target\\General.lvlib\\MFC SP"(w736) -> (error out=w734:errorcluster)  [unwired: 1 in]
      }
      event "bypass", "filter": Value Change {
        n352 = event-data() -> ()  [unwired: 1 in, 1 out]
        n353 = case shown="True" "bypass" {
          tunnel: [T23."Enabled" ("Disabled") T23."Disabled and Grayed Out" ("Disabled")] -> w752
          tunnel: [w756 w758] -> w751
          tunnel: "filter" -> [w755 _]
          frame False {
            n354 = Not(x=w755) -> (.not. x?=w754:bool)
            n355 = Build Array(w755, w754) -> (w756:bool[])
          }
          frame True {
            w759 = TRUE
            n356 = Build Array(w759, w759) -> (w758:bool[])
          }
        }
        n357 = property on="filter" class="Bool (strict)"("DisabledEnum"=w752) -> (error out=w749:errorcluster)  [unwired: 2 in, 1 out]
        n358 = shared-variable "RT PXI Target\\General.lvlib\\filterW"(w751, error in=w749) -> (error out=w748:errorcluster)
      }
      event "log_lin": Value Change {
        n359 = event-data() -> ()  [unwired: 1 in, 1 out]
        n360 = Boolean To (0,1)(Boolean="log_lin") -> (0, 1=w763:i16)
        n361 = To Unsigned Byte Integer(number=w763) -> (unsigned 8bit integer=w762:u8)
        n362 = property on="micFreq" class="WFGraph (strict)"("YScale.Mapping Mode"=w762) -> (error out=w761:errorcluster)  [unwired: 2 in, 1 out]
      }
      event "ACpow": Value Change {
        n363 = event-data() -> ()  [unwired: 1 in, 1 out]
        n364 = Cluster To Array(cluster="ACpow") -> (array=w765:bool[])
        n365 = shared-variable "RT PXI Target\\General.lvlib\\ACPow"(w765) -> (error out=w767:errorcluster)  [unwired: 1 in]
      }
      event "swDispl": Value Change {
        # "When the display is switched, reset the buttons that were previously true to false."
        n366 = event-data() -> ("NewVal"=w774:T1, "OldVal"=w775:T1)  [unwired: 1 in]
        n367 = Cluster To Array(cluster=w775) -> (array=w772:bool[])
        n368 = Cluster To Array(cluster=w774) -> (array=w771:bool[])
        n369 = Equal?(x=w771, y=w772) -> (x = y?=w773:bool[])
        n370 = for {
          tunnel: w773 -> [w780] mode=indexing
          tunnel: w772 -> [w779] mode=indexing
          tunnel: [w778] -> w770 mode=indexing
          tunnel: w771 -> [w777] mode=indexing
          i -> [w776]
          n371 = case shown="False" w780 {
            tunnel: w779 -> [_ w785]
            tunnel: [w782 w784] -> w778
            tunnel: w777 -> [w782 w783]
            tunnel: w776 -> [w781 _]
            frame False {
              n372 = local write "tabCtl"(w781) -> ()
            }
            frame True {
              n373 = case shown="False" w785 {
                tunnel: [w786 FALSE] -> w784
                tunnel: w783 -> [w786 _]
                frame False {
                }
                frame True {
                }
              }
            }
          }
        }
        n374 = Array To Cluster(array=w770) -> (cluster=w769:T44)
        n375 = local write "swDispl"(w769) -> ()
      }
    }
    n376 = call <userlib>:"checkForError.vi"("Error In"=w484) -> ()  [unwired: 9 in, 2 out]
  }
  n377 = call <vilib>:"Simple Error Handler.vi"("error in (no error)"=w3) -> ("error out"=w10:errorcluster)  [unwired: 4 in, 4 out]
  n378 = Open Application Reference(8:w10) -> (0:w12:errorcluster, 3:w11:refnum<vi>)  [unwired: 3 in]
  n379 = property class="App"(reference=w11, error in=w12) -> (reference out=w16:refnum<vi>, error out=w15:errorcluster, "App.Kind"=w14:T22)
  n380 = Equal?(x=w14, y=T22."Run Time System" ("Application:Kind")) -> (x = y?=w9:bool)
  n381 = Close Reference(reference=w16, error in (no error)=w15) -> ()  [unwired: 1 out]
  n382 = Quit LabVIEW(quit? (T)=w9) -> ()
